vi "Test DC Couple.vi"(8 "error in (no error)":errorcluster, 11 "SR7270 Drivers in":refnum<class "SR7270 Drivers.lvclass">) -> (0 "error out":errorcluster, 3 "SR7270 Drivers out":refnum<class "SR7270 Drivers.lvclass">)   [LabVIEW 2016, in "SR7270 Drivers.lvlib"]
uses:
  SR7270 Drivers.lvlib
  <vilib>/addons/_JKI Toolkits/Caraya/classes/Assert/Assert.lvclass
  <vilib>/addons/_JKI Toolkits/Caraya/classes/Test/Test.lvclass
  Typedefs/DCCOUPLE--enum.ctl
  SR7270 Drivers.lvclass
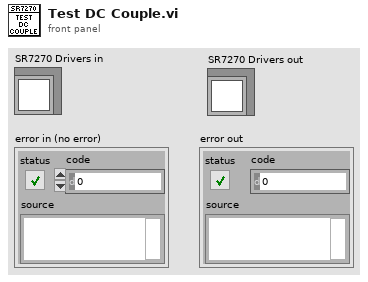
[diagram p1: front panel]
types:
  T1 = typedef "SR7270 Drivers.lvlib/DCCOUPLE--enum.ctl" = enum16{"AC coupled", "DC coupled"}
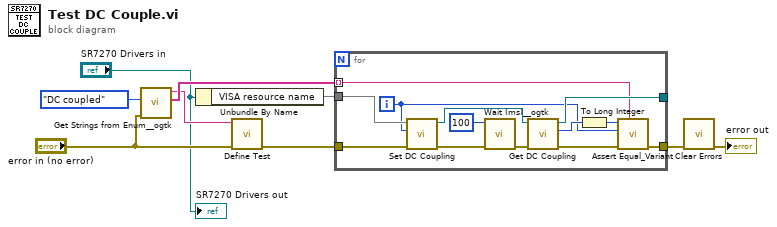
[diagram p0: block diagram]
diagram:
  n1 = call <userlib>:"Get Strings from Enum__ogtk.vi"("error in (no error)"="error in (no error)", "Enum"=DCCOUPLE--enum."DC coupled" ("DC Coupling")) -> ("Enum Strings"=w5:string[], "Enum Name"=w4:string)  [unwired: 6 in, 2 out]
  n2 = Unbundle By Name("SR7270 Drivers in") -> ("VISA resource name"=w2)
  n3 = call <vilib>:"Define Test.vi"("error in (no error)"="error in (no error)", "Label (VI Title)"=w4) -> ("error out"=w9:errorcluster)  [unwired: 9 in]
  n4 = for {
    tunnel: w2 -> [w21]
    tunnel: w9 -> [w13]
    tunnel: [w19] -> w8
    tunnel: [w18] -> _
    tunnel: w5 -> [w10] mode=indexing
    i -> [w12]
    n5 = call "Set DC Coupling.vi"("error in (no error)"=w13, "DC Coupling"=w12, "VISA resource name"=w21) -> ("error out"=w15:errorcluster, "VISA resource name out"=w22:refnum<visa-resource-name>)  [unwired: 7 in]
    n6 = call <userlib>:"Wait (ms)__ogtk.vi"("error in (no error)"=w15, "milliseconds to wait"=u32 100) -> ("error out"=w17:errorcluster)  [unwired: 8 in, 1 out]
    n7 = call "Get DC Coupling.vi"("error in (no error)"=w17, "VISA resource name"=w22) -> ("error out"=w20:errorcluster, "DC Coupling"=w14:T1, "VISA resource name out"=w18:refnum<visa-resource-name>)  [unwired: 7 in]
    n8 = To Long Integer(number=w14) -> (32bit integer=w11:i32)
    n9 = call <vilib>:"Assert Equal_Variant.vi"("Label"=w10, "error in (no error)"=w20, "Y"=w12, "X"=w11) -> ("error out"=w19:errorcluster)  [unwired: 7 in]
  }
  n10 = call <vilib>:"Clear Errors.vi"("error in (no error)"=w8) -> ("error out"=→"error out":errorcluster)  [unwired: 5 in, 1 out]
  "SR7270 Drivers out" <- "SR7270 Drivers in"
